vi "Send and Receive.vi"(7 "pre-read delay":i16=-1, 8 "error in (no error)":errorcluster, 9 "Termination Char":T1=enum."\\r\\n", 10 "data":string, 11 "Serial Base in":refnum<class "Serial Base.lvclass">) -> (0 "error out":errorcluster, 1 "bytes received":u32, 2 "buffer output":string, 3 "Serial Base out":refnum<class "Serial Base.lvclass">, 4 "bytes sent":u32)   [LabVIEW 2022 SP3, in "Serial-Com-Libraries.lvlib" / "Serial Base.lvclass"]
uses:
  Serial Base.lvclass
  Termination Character--enum.ctl
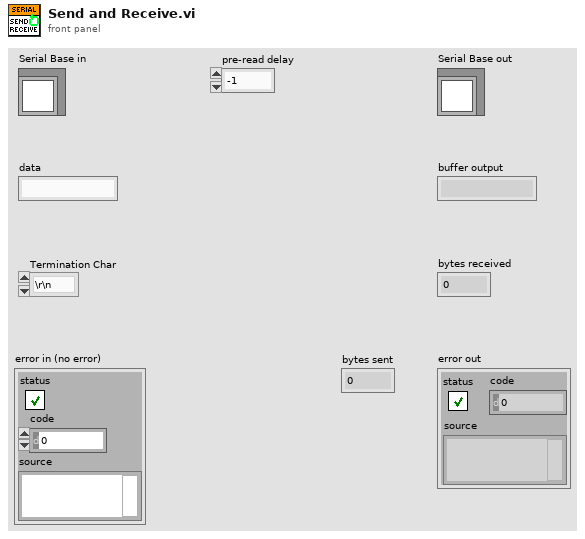
[diagram p1: front panel]
types:
  T1 = typedef "Serial-Com-Libraries.lvlib/Serial Base.lvclass/Termination Character--enum.ctl" = enum16{"none", "\\r\\n", "\\r", "\\n"}
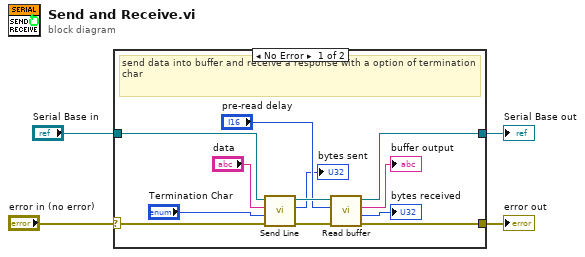
[diagram p0: block diagram]
diagram:
  n1 = case shown="No Error" "error in (no error)" {
    selector: "error in (no error)" -> [w9 w18]
    tunnel: [w7 w18] -> w3
    tunnel: [w14 w17] -> w1
    tunnel: "Serial Base in" -> [w16 w17]
    frame No Error {
      # "send data into buffer and receive a response with a option of termination char"
      n2 = call-dynamic "Send Line.vi"("error in (no error)"=w9, "Termination Char"="Termination Char", "data"="data", "Serial Base in"=w16) -> ("error out"=w8:errorcluster, "bytes count"=→"bytes sent":u32, "Serial Base out"=w15:refnum<class "Serial Base.lvclass">)  [unwired: 5 in]
      n3 = call-dynamic "Read buffer.vi"("error in (no error)"=w8, "pre-read delay"="pre-read delay", "Serial Base in"=w15) -> ("error out"=w7:errorcluster, "return count"=→"bytes received":u32, "buffer output"=→"buffer output":string, "Serial Base out"=w14:refnum<class "Serial Base.lvclass">)  [unwired: 5 in]
    }
    frame Error {
    }
  }
  "error out" <- w3
  "Serial Base out" <- w1
